vi "Not Supported on 32-Bit Systems.vi"   [LabVIEW 2020, in "common.lvlib"]
uses:
  common.lvlib
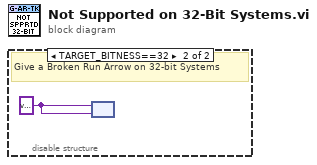
[diagram p0: block diagram]
diagram:
  n1 = disable-structure shown="TARGET_BITNESS==32" {
    frame condition #0 {
      # "Not 32-Bit - All Good"
    }
    frame condition #1 (active) {
      w1 = variant ("type")
      # "Give a Broken Run Arrow on 32-bit Systems"
      n2 = node(w1, w1) -> ()  [unwired: 1 out]
    }
  }
